vi "Circle.vi"(8 "error in (no error)":errorcluster, 10 "target":refnum<class "pCircle.lvclass">, 11 "pCircle in":refnum<class "pCircle.lvclass">) -> (0 "error out":errorcluster, 3 "pCircle out":refnum<class "pCircle.lvclass">)   [LabVIEW 2018, in "pCircle.lvclass"]
uses:
  pCircle.lvclass
  C:/Users/fflores/Documents/LabVIEW-Open-Projects/LabIVEW OOP Design Patterns/Prototype Pattern/Shape Class/pShape.lvclass
  pCircle.lvclass/pCircle.ctl
  Shape Class/pShape.lvclass
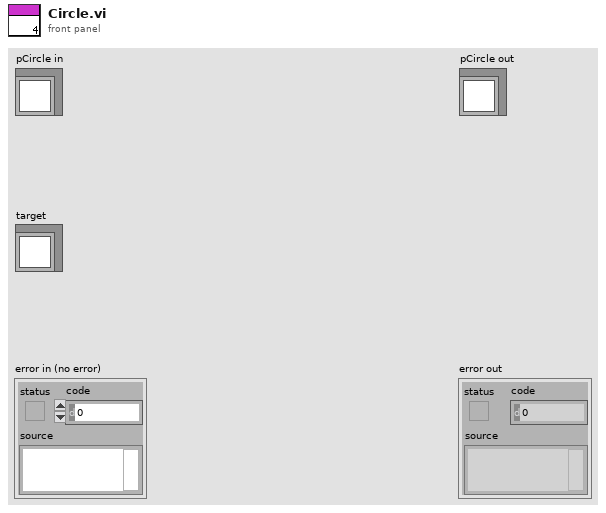
[diagram p1: front panel]
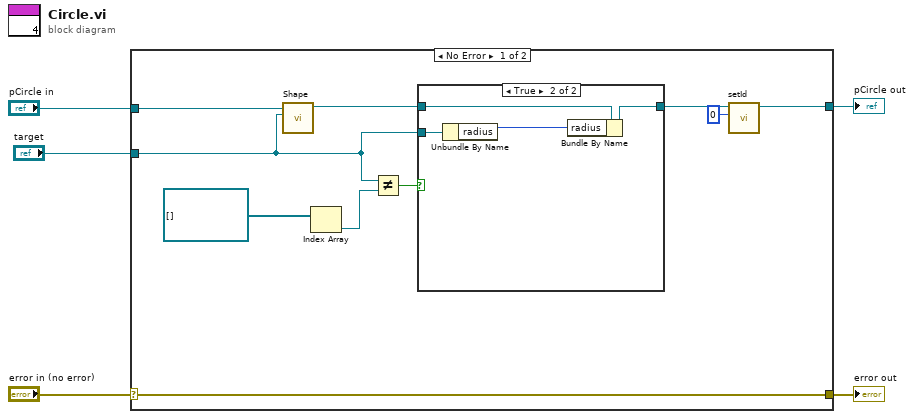
[diagram p0: block diagram]
diagram:
  n1 = case shown="No Error" "error in (no error)" {
    selector: "error in (no error)" -> [w15 w21]
    tunnel: [w15 w21] -> w4
    tunnel: [w7 w22] -> w2
    tunnel: "pCircle in" -> [w12 w22]
    tunnel: "target" -> [w9 _]
    frame No Error {
      n2 = call "Shape.vi"("pShape.lvclass"=w9, "pShape in"=w12) -> ("pShape out"=w10:refnum<class "pCircle.lvclass">)  [unwired: 8 in, 1 out]
      n3 = Index Array(array=refnum<class "pCircle.lvclass">[] []) -> (element=w14:refnum<class "pCircle.lvclass">)  [unwired: 1 in]
      n4 = Not Equal?(x=w9, y=w14) -> (x != y?=w8:bool)
      n5 = case shown="True" w8 {
        tunnel: [w16 w20] -> w11
        tunnel: w10 -> [w16 w19]
        tunnel: w9 -> [_ w18]
        frame False {
        }
        frame True {
          n6 = Unbundle By Name(w18) -> ("radius"=w17:i32)
          n7 = Bundle By Name(cluster=w19, "radius"=w17) -> (w20:refnum<class "pCircle.lvclass">)
        }
      }
      n8 = call-dynamic "setId.vi"("ID"=0, "pCircle in"=w11) -> ("pCircle out"=w7:refnum<class "pCircle.lvclass">)  [unwired: 8 in, 1 out]
    }
    frame Error {
      # "Wire the error cluster across even in the \"No Error\"\ncase so that warnings get propagated."
    }
  }
  "error out" <- w4
  "pCircle out" <- w2
